vi "Update.vi"(8 "error in (no error)":errorcluster, 11 "senseHatJoystick in":refnum<class "RPI.SenseHat.Joystick.lvclass">) -> (0 "error out":errorcluster, 2 "Joystick":T1, 3 "senseHatJoystick out":refnum<class "RPI.SenseHat.Joystick.lvclass">)   [LabVIEW 2020, in "RPI.SenseHat.Joystick.lvlib" / "RPI.SenseHat.Joystick.lvclass"]
uses:
  RPI.SenseHat.Joystick.lvclass
  TypeDefs/Joystick.ctl
  RPI.SenseHat.Joystick.lvclass/RPI.SenseHat.Joystick.ctl
  RPI/Classes/mainI2CDevice/mainI2CDevice.lvclass
  RPI.SenseHat.Joystick.lvlib
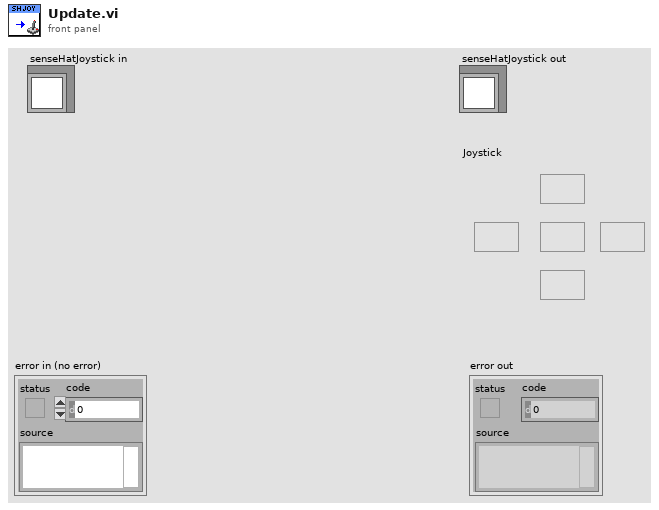
[diagram p1: front panel]
types:
  T1 = typedef "RPI.SenseHat.Joystick.lvlib/Joystick.ctl" = cluster{"Enter":bool, "Down":bool, "Up":bool, "Right":bool, "Left":bool}
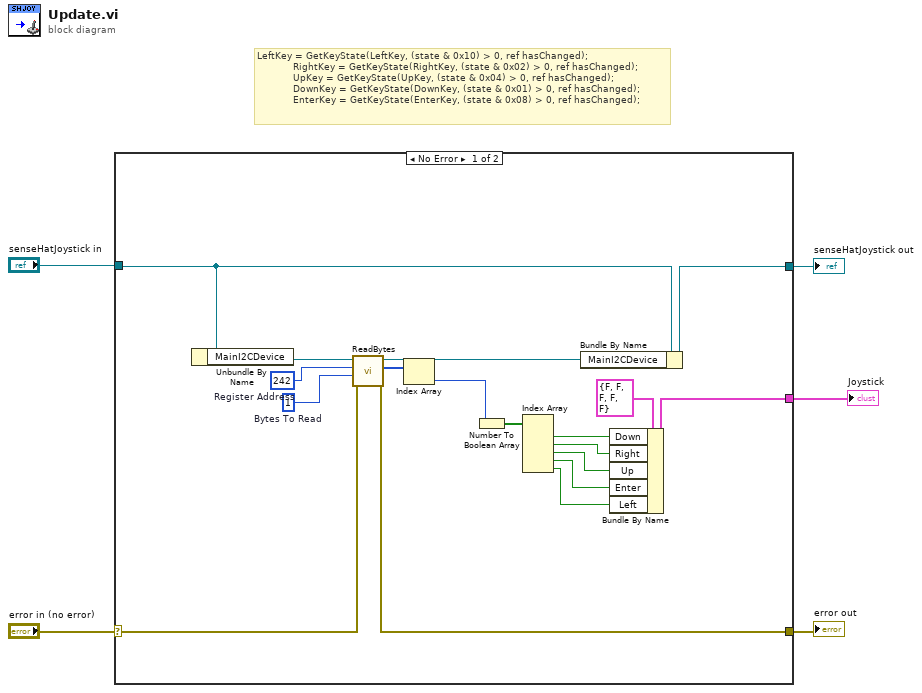
[diagram p0: block diagram]
diagram:
  # "LeftKey = GetKeyState(LeftKey, (state & 0x10) > 0, ref hasChanged);\n            RightKey = GetKeyState(RightKey, (state & 0x02) > 0, ref hasChanged);\n            UpKey = GetKeyState(UpKey, (state & 0x04) > 0, ref hasChanged);\n            DownKey = GetKeyState(DownKey, (state & 0x01) > 0, ref hasChanged);\n            EnterKey = GetKeyState(EnterKey, (state & 0x08) > 0, ref hasChanged);"
  n1 = case shown="No Error" "error in (no error)" {
    selector: "error in (no error)" -> [w19 w25]
    tunnel: [w18 w25] -> w4
    tunnel: [w22 w24] -> w2
    tunnel: "senseHatJoystick in" -> [w23 w24]
    tunnel: [w11 _] -> w1
    frame No Error {
      w16 = u8 242  # Register Address
      w17 = u8 1  # Bytes To Read
      n2 = Unbundle By Name(w23) -> ("MainI2CDevice"=w21:refnum<class "mainI2CDevice.lvclass">)
      n3 = call "ReadBytes.vi"("error in (no error)"=w19, "Bytes To Read"=w17, "Register Address"=w16, "mainI2CDevice in"=w21) -> ("error out"=w18:errorcluster, "Data"=w15:u8[], "mainI2CDevice out"=w20:refnum<class "mainI2CDevice.lvclass">)  [unwired: 5 in]
      n4 = Index Array(array=w15) -> (element=w14:u8)  [unwired: 1 in]
      n5 = Number To Boolean Array(number=w14) -> (Boolean array=w13:bool[])
      n6 = Index Array(array=w13) -> (element #1=w10:bool, element #2=w9:bool, element #3=w8:bool, element #4=w7:bool, element #5=w6:bool)  [unwired: 5 in]
      n7 = Bundle By Name(cluster=w23, "MainI2CDevice"=w20) -> (w22:refnum<class "RPI.SenseHat.Joystick.lvclass">)
      n8 = Bundle By Name(cluster=T1 {"Enter"=FALSE, "Down"=FALSE, "Up"=FALSE, "Right"=FALSE, "Left"=FALSE} ("Joystick"), "Down"=w10, "Right"=w9, "Up"=w8, "Enter"=w7, "Left"=w6) -> (w11:T1)
    }
    frame Error {
    }
  }
  "error out" <- w4
  "senseHatJoystick out" <- w2
  "Joystick" <- w1
